vi "AddLogo.vi"(8 "图片尺寸":cluster{"right":i16, "bottom":i16}={"right"=176, "bottom"=176}, 9 "logo尺寸":T1={"left"=0, "top"=0, "right"=64, "bottom"=64}, 11 "图片输入":picture) -> (0 "error out":errorcluster caption="错误输出", 3 "图片输出":picture)   [LabVIEW 2016]
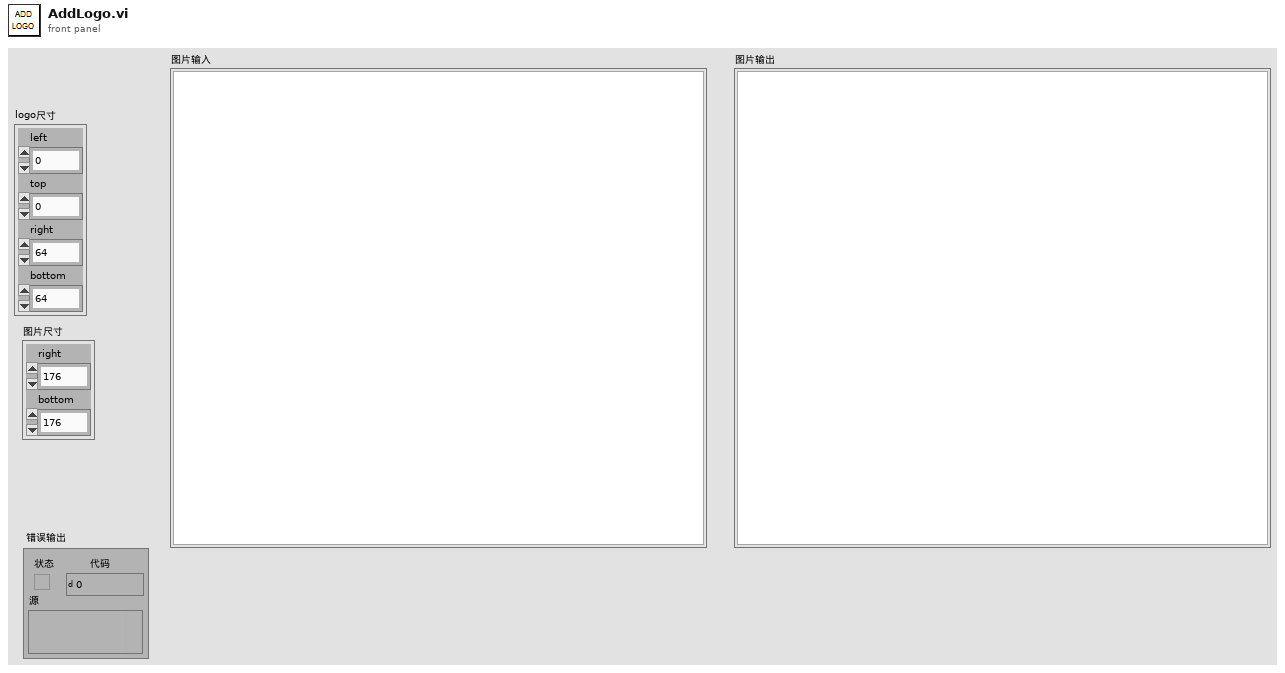
[diagram p1: front panel]
types:
  T1 = cluster{"left":i16, "top":i16, "right":i16, "bottom":i16}
  T2 = typedef "imagedata.ctl" = cluster{"image type":i32, "image depth":i32, "image":u8[], "mask":u8[], "colors":u32[], "Rectangle":cluster{"left":i16, "top":i16, "right":i16, "bottom":i16}}
  T3 = cluster{"image[0]":u8, "image[1]":u8, "image[2]":u8}
  T4 = cluster{"Width":u16, "Style":enum32{"Solid", "Dash", "Dot", "DashDot", "DashDotDot"}}
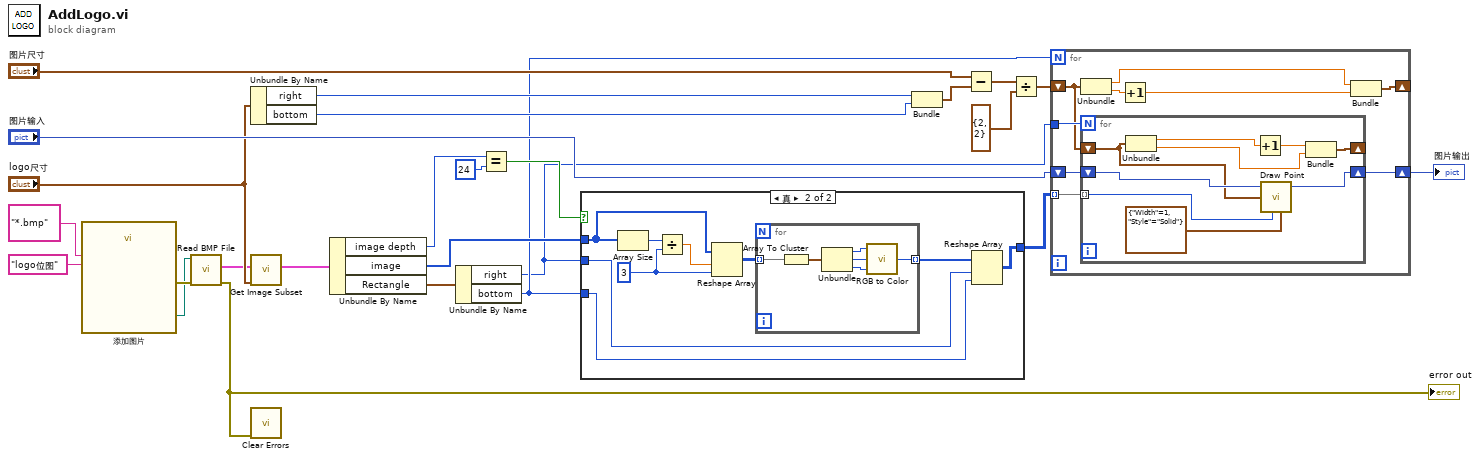
[diagram p0: block diagram]
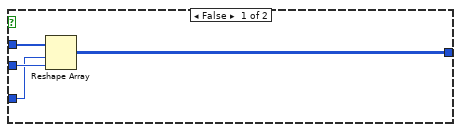
[diagram p2: hidden frame]
diagram:
  n1 = call "添加图片"("pattern (all files)"="*.bmp", "pattern label"="logo位图") -> ("selected path"=w3:path, "error out"=w4:errorcluster)  [unwired: 10 in, 2 out]
  n2 = call <vilib>:"Read BMP File.vi"("error in (no error)"=w4, "path to BMP file"=w3) -> ("error out"=w1:errorcluster, "image data"=w6:T2)  [unwired: 7 in, 1 out]
  "error out" <- w1
  n3 = Unbundle By Name("logo尺寸") -> ("right"=w19:i16, "bottom"=w18:i16)
  n4 = call <vilib>:"Get Image Subset.vi"("subset rect"="logo尺寸", "image data"=w6) -> ("image subset"=w11:T2)  [unwired: 4 in, 1 out]
  n5 = call <vilib>:"Clear Errors.vi"("error in (no error)"=w1) -> ()  [unwired: 5 in, 2 out]
  n6 = Unbundle By Name(w11) -> ("image depth"=w15:i32, "image"=w12:u8[], "Rectangle"=w24:T1)
  n7 = Unbundle By Name(w24) -> ("right"=w8:i16, "bottom"=w9:i16)
  n8 = Equal?(x=w15, y=24) -> (x = y?=w13:bool)
  n9 = case shown="真" w13 {
    tunnel: w12 -> [w29 w38]
    tunnel: [w27 w32] -> w10
    tunnel: w9 -> [w26 w31]
    tunnel: w8 -> [w28 w30]
    frame False {
      n10 = Reshape Array(w29, w26, w28) -> (w27:u8[][])
    }
    frame True {
      w37 = 3 ("维数大小")
      n11 = Array Size(array=w38) -> (size(s)=w36:i32)
      n12 = Divide(x=w36, y=w37) -> (x/y=w35:dbl)
      n13 = Reshape Array(w38, w35, w37) -> (w34:u8[][])
      n14 = for {
        tunnel: w34 -> [w44] mode=indexing
        tunnel: [w39] -> w33 mode=indexing
        n15 = Array To Cluster(array=w44) -> (cluster=w43:T3)
        n16 = Unbundle(w43) -> ("image[0]"=w42:u8, "image[1]"=w41:u8, "image[2]"=w40:u8)
        n17 = call <vilib>:"RGB to Color.vi"("B"=w40, "G"=w41, "R"=w42) -> ("Color"=w39:u32)
      }
      n18 = Reshape Array(w33, w30, w31) -> (w32:u32[][])
    }
  }
  n19 = Bundle("right"=w19, "bottom"=w18) -> (w17:cluster{"right":i16, "bottom":i16})  [unwired: 1 in]
  n20 = Subtract(x="图片尺寸", y=w17) -> (x-y=w16:cluster{"right":i16, "bottom":i16})
  n21 = Divide(x=w16, y=cluster{"right":i16, "bottom":i16} {"right"=2, "bottom"=2}) -> (x/y=w7:cluster{"right":dbl, "bottom":dbl})
  n22 = for {
    N: w9 -> [_]
    tunnel: w8 -> [w53]
    shift-right: [w47] -> _
    shift-left: w7 -> [w48]
    shift-right: [w46] -> w25
    shift-left: "图片输入" -> [w52]
    tunnel: w10 -> [w45] mode=indexing
    n23 = Unbundle(w48) -> ("right"=w51:dbl, "bottom"=w50:dbl)
    n24 = for {
      N: w53 -> [_]
      shift-right: [w61] -> w46
      shift-left: w52 -> [w62]
      shift-right: [w56] -> _
      shift-left: w48 -> [w60]
      tunnel: w45 -> [w55] mode=indexing
      n25 = Unbundle(w60) -> ("right"=w58:dbl, "bottom"=w59:dbl)
      n26 = Increment(x=w58) -> (x+1=w57:dbl)
      n27 = call <vilib>:"Draw Point.vi"("picture"=w62, "point(x,y)"=w60, "color(black)"=w55, "pen"=T4 {"Width"=1, "Style"=enum."Solid"}) -> ("new picture"=w61:picture)  [unwired: 5 in]
      n28 = Bundle(w57, "bottom"=w59) -> (w56:cluster{dbl, "bottom":dbl})  [unwired: 1 in]
    }
    n29 = Increment(x=w50) -> (x+1=w49:dbl)
    n30 = Bundle("right"=w51, w49) -> (w47:cluster{"right":dbl, dbl})  [unwired: 1 in]
  }
  "图片输出" <- w25
